vi "Status String.vi"(6 "LabPack Shared Library":path=path "", 8 "Error In":errorcluster, 11 "Status":T1) -> (0 "Error Out":errorcluster, 3 "Text":string)   [LabVIEW 2019, in "LabPack.lvlib"]
doc: "Converts a LabPack shared library status to a more descriptive string."
uses:
  LabPack.lvlib
  Controls/Status.ctl
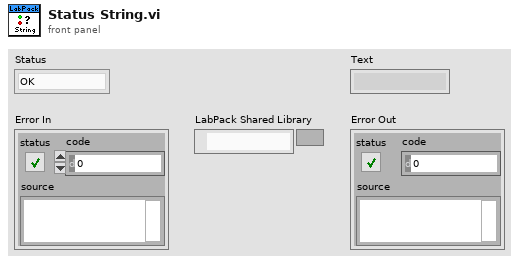
[diagram p1: front panel]
types:
  T1 = typedef "LabPack.lvlib/Status.ctl" = enum32{"OK", "Out of Memory", "Null Value", "Encoder", "Decoder"}
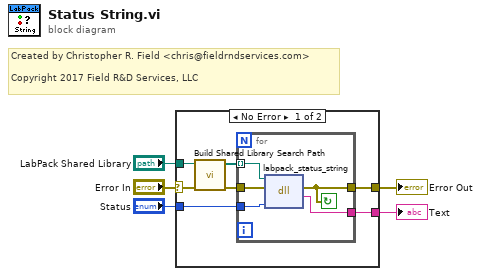
[diagram p0: block diagram]
diagram:
  # "Created by Christopher R. Field <chris@fieldrndservices.com>\n\nCopyright 2017 Field R&D Services, LLC"
  n1 = case shown="No Error" "Error In" {
    selector: "Error In" -> [w11 w18]
    tunnel: [w12 w18] -> w5
    tunnel: "LabPack Shared Library" -> [w8 _]
    tunnel: "Status" -> [w7 _]
    tunnel: [w6 _] -> w1
    frame No Error {
      n2 = call "Build Shared Library Search Path.vi"("Error In"=w11, "LabPack Shared Library"=w8) -> ("Error Out"=w10:errorcluster, "Search Path"=w9:path[])  [unwired: 8 in]
      n3 = for {
        tunnel: w9 -> [w16] mode=indexing
        tunnel: w10 -> [w17]
        tunnel: [w15] -> w12
        tunnel: w7 -> [w14]
        tunnel: [w13] -> w6
        stop <- w15 continue-if-true
        n4 = dll-call lib="D:/Users/cfield/Code/MessagePack/LabPack/LabVIEW/trunk/src/LabPack/Private/labpack-x64.dll" fn="labpack_status_string"(path in=w16, error in=w17, "status"=w14) -> (error out=w15:errorcluster, "return type"=w13:string)  [unwired: 2 in, 1 out]
      }
    }
    frame Error {
    }
  }
  "Error Out" <- w5
  "Text" <- w1
